vi "VLS.vi"(0 "System no.":i32=1 min=1 max=4 step=1, 3 "Velocity":dbl format="%.6f", 4 "No.of digits":i16=4, 5 "error in":errorcluster) -> (14 "Controller error":bool, 19 "error out":errorcluster)   [LabVIEW 2020]
doc: "Sets platform velocity and checks for error. Number of digits is the number of digits after the decimal point in the velocity value(s) that will be sent. Controller error is TRUE if selected system reports error code which is not 0.\n\nC-887, F-206, M-8X0: Only valid for GCS syntax version = GCS 2.0 or higher (check with CSV?.vi. If CSV?.vi is not supported, syntax version is GCS 1.0)."
panel:
  # "Sets platform velocity and \nchecks for error."
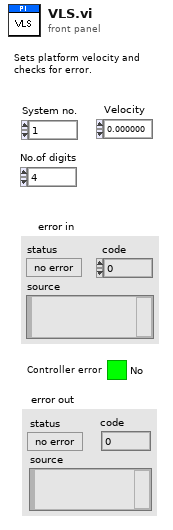
[diagram p1: front panel]
types:
  T1 = enum16{"Disable error check", "Force error check", "Use global settings"}
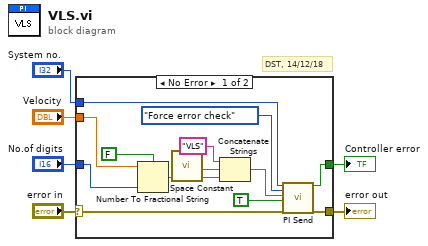
[diagram p0: block diagram]
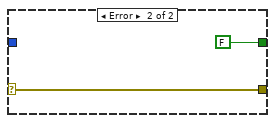
[diagram p2: hidden frame]
diagram:
  # "DST, 14/12/18"
  n1 = case shown="No Error" "error in" {
    selector: "error in" -> [w13 w21]
    tunnel: [w14 w21] -> w6
    tunnel: "Velocity" -> [w10 _]
    tunnel: "No.of digits" -> [w11 _]
    tunnel: "System no." -> [w19 _]
    tunnel: [w7 FALSE ("Controller error")] -> w1
    frame No Error {
      n2 = Number To Fractional String(use system decimal point (T)=FALSE, number=w10, precision (6)=w11) -> (F-format string=w8:string)  [unwired: 1 out]
      n3 = call "Space Constant.vi"() -> ("String"=w12:string)
      n4 = Concatenate Strings("VLS", w12, w8) -> (w17:string)
      n5 = call "PI Send.vi"("System no."=w19, "Error check settings"=T1."Force error check", "String to send"=w17, "Attach termination char.?"=TRUE ("Attach Linefeed?"), "error in"=w13) -> ("Controller error"=w7:bool, "error out"=w14:errorcluster)  [unwired: 1 in, 12 out]
    }
    frame Error {
    }
  }
  "error out" <- w6
  "Controller error" <- w1
